vi "Launch Test Engine Actor.vi"(8 "error in (no error)":errorcluster, 11 "TestBench in":refnum<class "TestBench.lvclass">) -> (0 "error out":errorcluster, 3 "TestBench out":refnum<class "TestBench.lvclass">)   [LabVIEW 2019, in "TestBench.lvlib" / "TestBench.lvclass"]
uses:
  TestBench.lvclass
  C:/Program Files (x86)/National Instruments/LabVIEW 2019/vi.lib/ActorFramework/Actor/Actor.lvclass
  TestBench.lvclass/TestBench.ctl
  UnitTestEngine/UnitTestEngine/UnitTestEngine.lvclass
  <vilib>/ActorFramework/Actor/Actor.lvclass/Actor.ctl
  <vilib>/ActorFramework/Message Enqueuer/Message Enqueuer.lvclass/Message Enqueuer.ctl
  UnitTestEngine/UnitTestEngine Messages/Change Windows Title Msg/Change Windows Title Msg.lvclass/Change Windows Title Msg.ctl
  41b1cc7d-7908-4545-958f-1a6c7b3a1be7.vi
  <vilib>/ActorFramework/Message Enqueuer/Init from Existing Queue.vi
  <vilib>/ActorFramework/Message Enqueuer/Enqueue.vi
  UnitTestEngine/UnitTestEngine Messages/Change Windows Title Msg/Change Windows Title Msg.lvclass
  C:/Program Files (x86)/National Instruments/LabVIEW 2019/vi.lib/ActorFramework/Message/Message.lvclass
  <vilib>/ActorFramework/Message Priority Queue/Priority Enqueue.vi
  <vilib>/ActorFramework/Message Enqueuer/Message Enqueuer.lvclass
  <vilib>/ActorFramework/Actor/Actor.lvclass
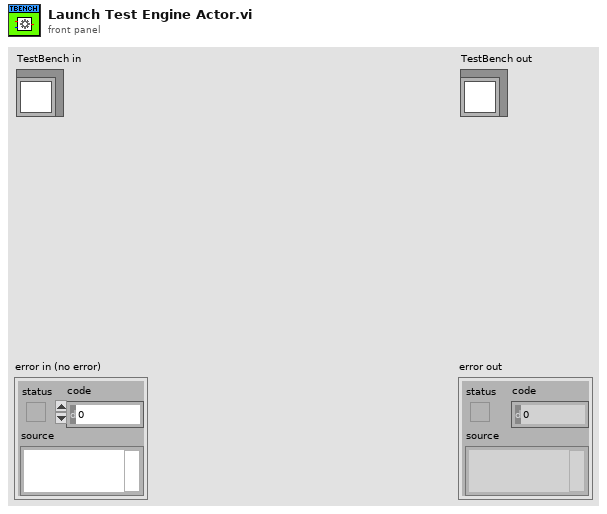
[diagram p1: front panel]
types:
  T1 = map{string, refnum<class "Message Enqueuer.lvclass">}
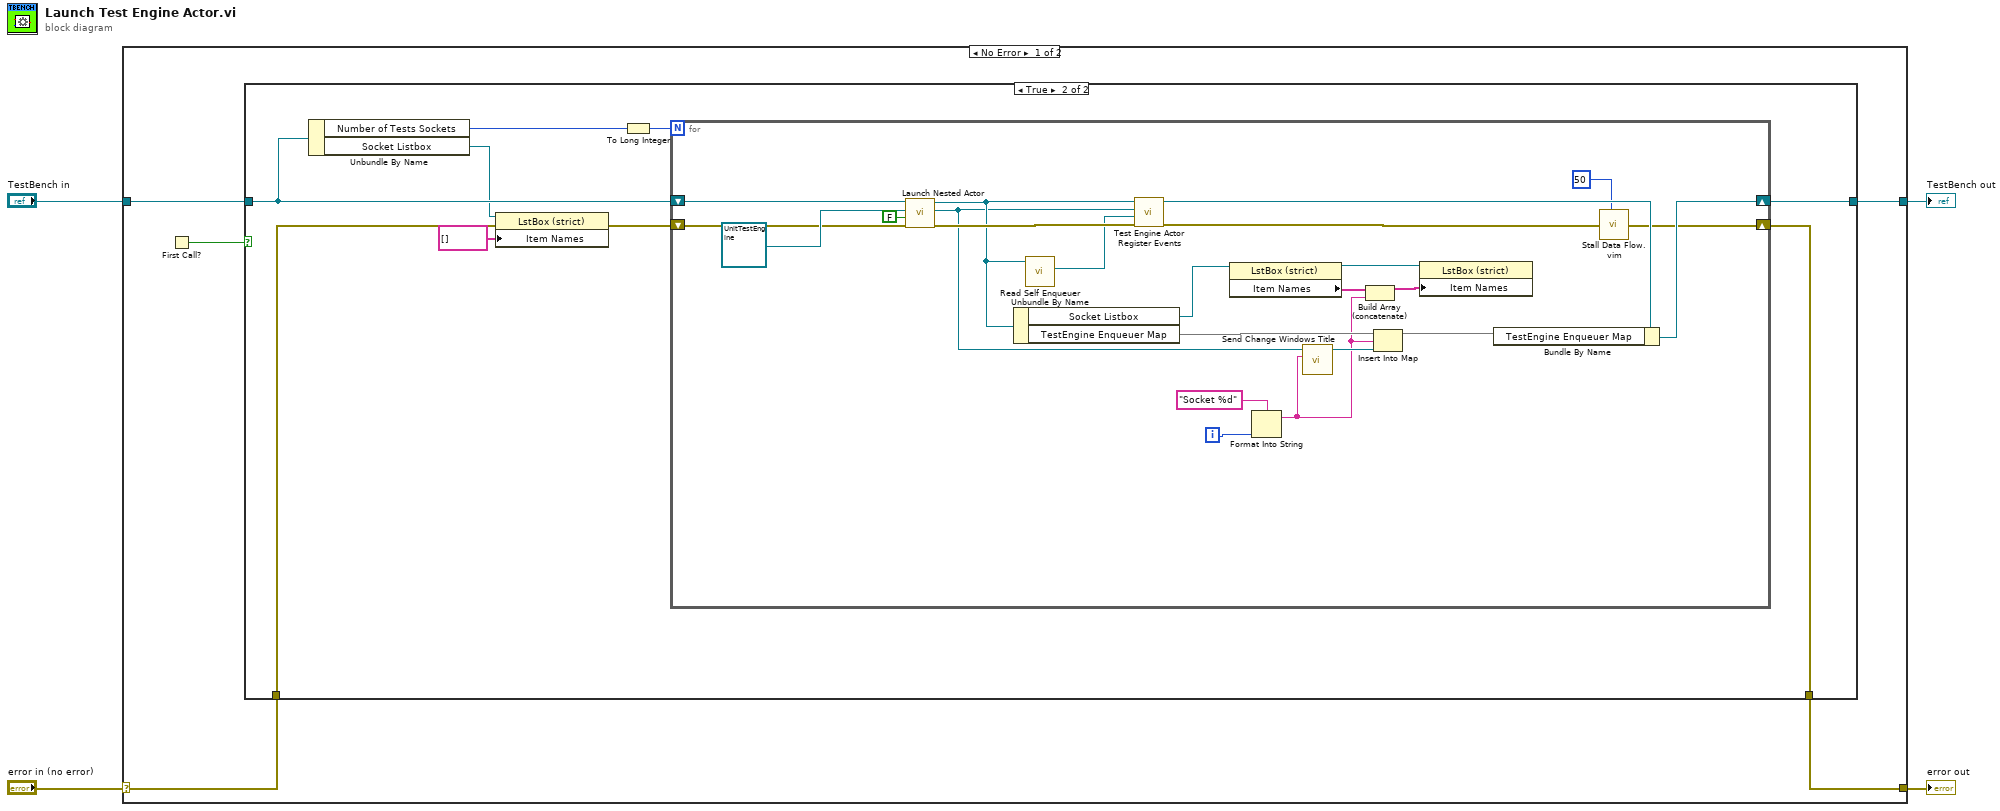
[diagram p0: block diagram]
diagram:
  n1 = case shown="No Error" "error in (no error)" {
    selector: "error in (no error)" -> [w7 w45]
    tunnel: [w8 w45] -> w3
    tunnel: [w9 w44] -> w1
    tunnel: "TestBench in" -> [w6 w44]
    frame No Error {
      n2 = First Call?() -> (First Call?: T/F=w5:bool)
      n3 = case shown="True" w5 {
        tunnel: [w11 w20] -> w9
        tunnel: [w10 w19] -> w8
        tunnel: w7 -> [w10 w14]
        tunnel: w6 -> [w11 w18]
        frame False {
        }
        frame True {
          n4 = Unbundle By Name(w18) -> ("Number of Tests Sockets"=w17:u8, "Socket Listbox"=w15:refnum<vi>)
          n5 = property class="LstBox (strict)"(reference=w15, error in=w14, "Item Names"=string[] []) -> (error out=w13:errorcluster)  [unwired: 1 out]
          n6 = To Long Integer(number=w17) -> (32bit integer=w16:i32)
          n7 = for {
            N: w16 -> [_]
            shift-right: [w26] -> w19
            shift-left: w13 -> [w38]
            shift-right: [w41] -> w20
            shift-left: w18 -> [w37]
            i -> [w36]
            n8 = call <vilib>:"Launch Nested Actor.vi"("error in (no error)"=w38, "Auto-stop? (T)"=FALSE, "Nested Actor"=refnum<class "UnitTestEngine.lvclass"> refnum ("UnitTestEngine.lvlib:UnitTestEngine.lvclass"), "Caller Actor in"=w37) -> ("error out"=w34:errorcluster, "Nested Actor's Enqueuer"=w23:refnum<class "Message Enqueuer.lvclass">, "Caller Actor out"=w32:refnum<class "TestBench.lvclass">)  [unwired: 5 in]
            n9 = Unbundle By Name(w32) -> ("Socket Listbox"=w30:refnum<vi>, "TestEngine Enqueuer Map"=w43:T1)
            n10 = call <vilib>:"Read Self Enqueuer.vi"("Actor"=w32) -> ("Self Enqueuer"=w31:refnum<class "Message Enqueuer.lvclass">)  [unwired: 10 in]
            n11 = call "Test Engine Actor Register Events.vi"("error in (no error)"=w34, "Registrant Address"=w31, "Event Source Address"=w23, "TestBench in"=w32) -> ("error out"=w33:errorcluster, "TestBench out"=w35:refnum<class "TestBench.lvclass">)  [unwired: 6 in]
            n12 = property class="LstBox (strict)"(reference=w30) -> (reference out=w29:refnum<vi>, "Item Names"=w28:string[])  [unwired: 1 in, 1 out]
            n13 = Format Into String(format string="Socket %d", w36) -> (resulting string=w21:string)  [unwired: 2 in, 1 out]
            n14 = call "Send Change Windows Title.vi"("Front Panel Window:Title"=w21, "Message Enqueuer"=w23) -> ("Message Enqueuer out"=w22:refnum<class "Message Enqueuer.lvclass">)  [unwired: 8 in, 1 out]
            n15 = Build Array (concatenate)(w28, w21) -> (w27:string[])
            n16 = Insert Into Map(map in=w43, key=w21, value=w22) -> (map out=w42:T1)  [unwired: 2 out]
            n17 = property class="LstBox (strict)"(reference=w29, "Item Names"=w27) -> ()  [unwired: 1 in, 2 out]
            n18 = Bundle By Name(cluster=w35, "TestEngine Enqueuer Map"=w42) -> (w41:refnum<class "TestBench.lvclass">)
            n19 = call "Stall Data Flow.vim"("value in"=w33, "milliseconds to wait"=u32 50) -> ("value out"=w26:errorcluster)  [unwired: 1 out]
          }
        }
      }
    }
    frame Error {
    }
  }
  "error out" <- w3
  "TestBench out" <- w1
